vi "Queue Comms FG.vi"(8 "error in":errorcluster, 10 "Action":T1, 11 "Queue in":refnum<queue>) -> (0 "error out":errorcluster, 3 "Queue out":refnum<queue>)   [LabVIEW 2010, in "Display Console.lvlib"]
doc: "This VI is a FG that provides access to the queue for the module."
uses:
  Display Console.lvlib
  Private Controls/Display Action.ctl
  Private Controls/Module Data Cluster.ctl
  Private Controls/Queue FG Action.ctl
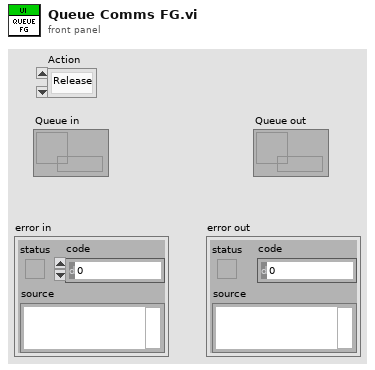
[diagram p1: front panel]
types:
  T1 = typedef "Display Console.lvlib/Queue FG Action.ctl" = enum16{"Release", "Get", "Set"}
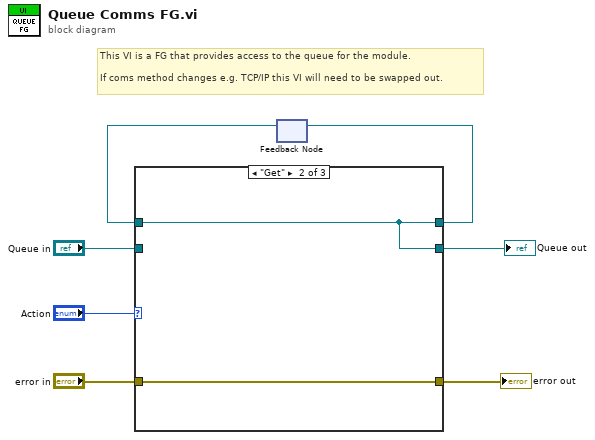
[diagram p0: block diagram]
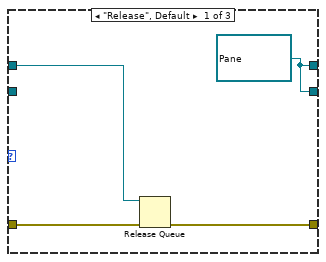
[diagram p2: hidden frame]
diagram:
  # "This VI is a FG that provides access to the queue for the module.\n\nIf coms method changes e.g. TCP/IP this VI will need to be swapped out."
  n1 = feedback #1() -> (w5:refnum<queue>)  [unwired: 1 in]
  n2 = case shown="\"Get\"" "Action" {
    tunnel: "Queue in" -> [_ _ w15]
    tunnel: [w8 w13 w15] -> w3
    tunnel: w5 -> [w11 w13 _]
    tunnel: [w8 w13 w15] -> w4
    tunnel: "error in" -> [w10 w12 w14]
    tunnel: [w9 w12 w14] -> w1
    frame "Release", Default {
      w8 = refnum<queue> refnum ("Queue in")
      n3 = Release Queue(queue=w11, error in (no error)=w10) -> (error out=w9:errorcluster)  [unwired: 1 in, 2 out]
    }
    frame "Get" {
    }
    frame "Set" {
    }
  }
  "Queue out" <- w3
  "error out" <- w1
  n4 = feedback-in #1(w4) -> ()
